vi "Set AddRun Controls Values.vi"(7 "Subpanels Map":map{string, refnum<vi>}(c390), 8 "error in":errorcluster, 11 "Schedule Block":refnum<class "Schedule Block.lvclass">) -> (0 "error out":errorcluster, 2 "Script Path":path, 4 "SubPanel VI out":refnum<vi>)   [LabVIEW 2020, in "TALOS.lvlib" / "Scheduler.lvlib"]
uses:
  Scheduler.lvlib
  Run Utilities/Schedule Block/Schedule Block.lvclass
  Add RUN Window.vi
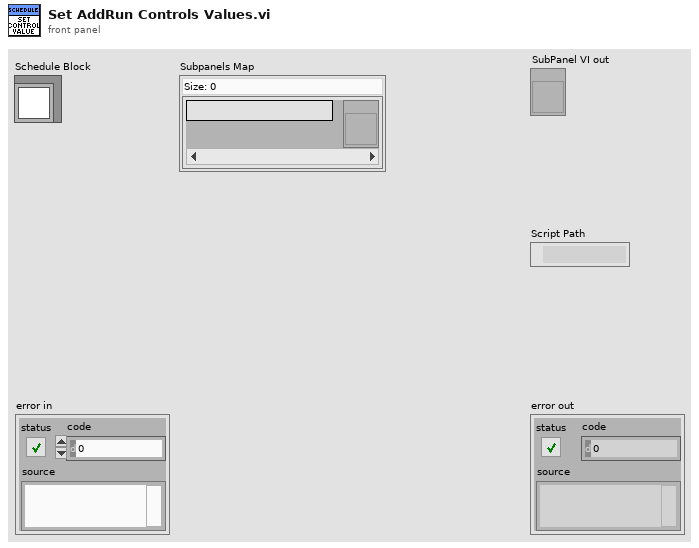
[diagram p1: front panel]
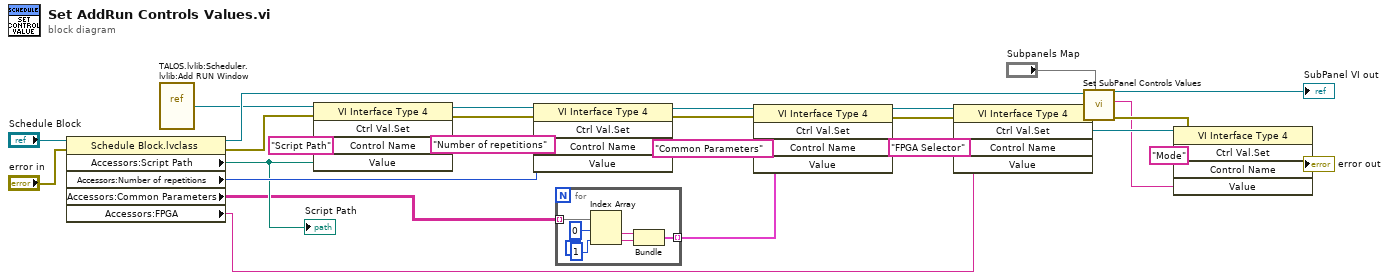
[diagram p0: block diagram]
diagram:
  n1 = property class="Schedule Block.lvclass"(reference="Schedule Block", error in="error in") -> (reference out=w11:refnum<class "Schedule Block.lvclass">, error out=w16:errorcluster, "Accessors:Script Path"=w18:path, "Accessors:Number of repetitions"=w19:u16, "Accessors:Common Parameters"=w15:string[][], "Accessors:FPGA"=w4:string)
  "Script Path" <- w18
  n2 = vi-ref "TALOS.lvlib:Scheduler.lvlib:Add RUN Window.vi"() -> (w3:refnum<vi>)
  n3 = invoke class="VI Interface Type 4" method="Ctrl Val.Set"(reference=w3, error in=w16, "Control Name"="Script Path", "Value"=w18) -> (reference out=w26:refnum<vi>, error out=w25:errorcluster)  [unwired: 1 in, 3 out]
  n4 = invoke class="VI Interface Type 4" method="Ctrl Val.Set"(reference=w26, error in=w25, "Control Name"="Number of repetitions", "Value"=w19) -> (reference out=w21:refnum<vi>, error out=w20:errorcluster)  [unwired: 1 in, 3 out]
  n5 = for {
    tunnel: w15 -> [w34] mode=indexing
    tunnel: [w29] -> w14 mode=indexing
    n6 = Index Array(array=w34, index #1=0 ("index"), index #2=1 ("index")) -> (element #1=w31:string, element #2=w30:string)
    n7 = Bundle("String"=w31, "String"=w30) -> (w29:cluster{"String":string, "String":string})  [unwired: 1 in]
  }
  n8 = invoke class="VI Interface Type 4" method="Ctrl Val.Set"(reference=w21, error in=w20, "Control Name"="Common Parameters", "Value"=w14) -> (reference out=w9:refnum<vi>, error out=w8:errorcluster)  [unwired: 1 in, 3 out]
  n9 = invoke class="VI Interface Type 4" method="Ctrl Val.Set"(reference=w9, error in=w8, "Control Name"="FPGA Selector", "Value"=w4) -> (reference out=w6:refnum<vi>, error out=w7:errorcluster)  [unwired: 1 in, 3 out]
  n10 = call "Set SubPanel Controls Values.vi"("Subpanels Map"="Subpanels Map", "error in (no error)"=w7, "Schedule Block in"=w11) -> ("error out"=w28:errorcluster, "SBlock Type"=w2:string, "SubPanel VI out"=→"SubPanel VI out":refnum<vi>)  [unwired: 6 in]
  n11 = invoke class="VI Interface Type 4" method="Ctrl Val.Set"(reference=w6, error in=w28, "Control Name"="Mode", "Value"=w2) -> (error out=→"error out":errorcluster)  [unwired: 1 in, 4 out]
